vi "Terminal_Global_Pressure_system.vi"() -> ()   [LabVIEW 2014]
panel:
  out "试验单元监测参数":T1
  out "陪试单元监测参数":T2
  out "加载单元监测参数":T3
  # "报警信息"
  # "报警信息"
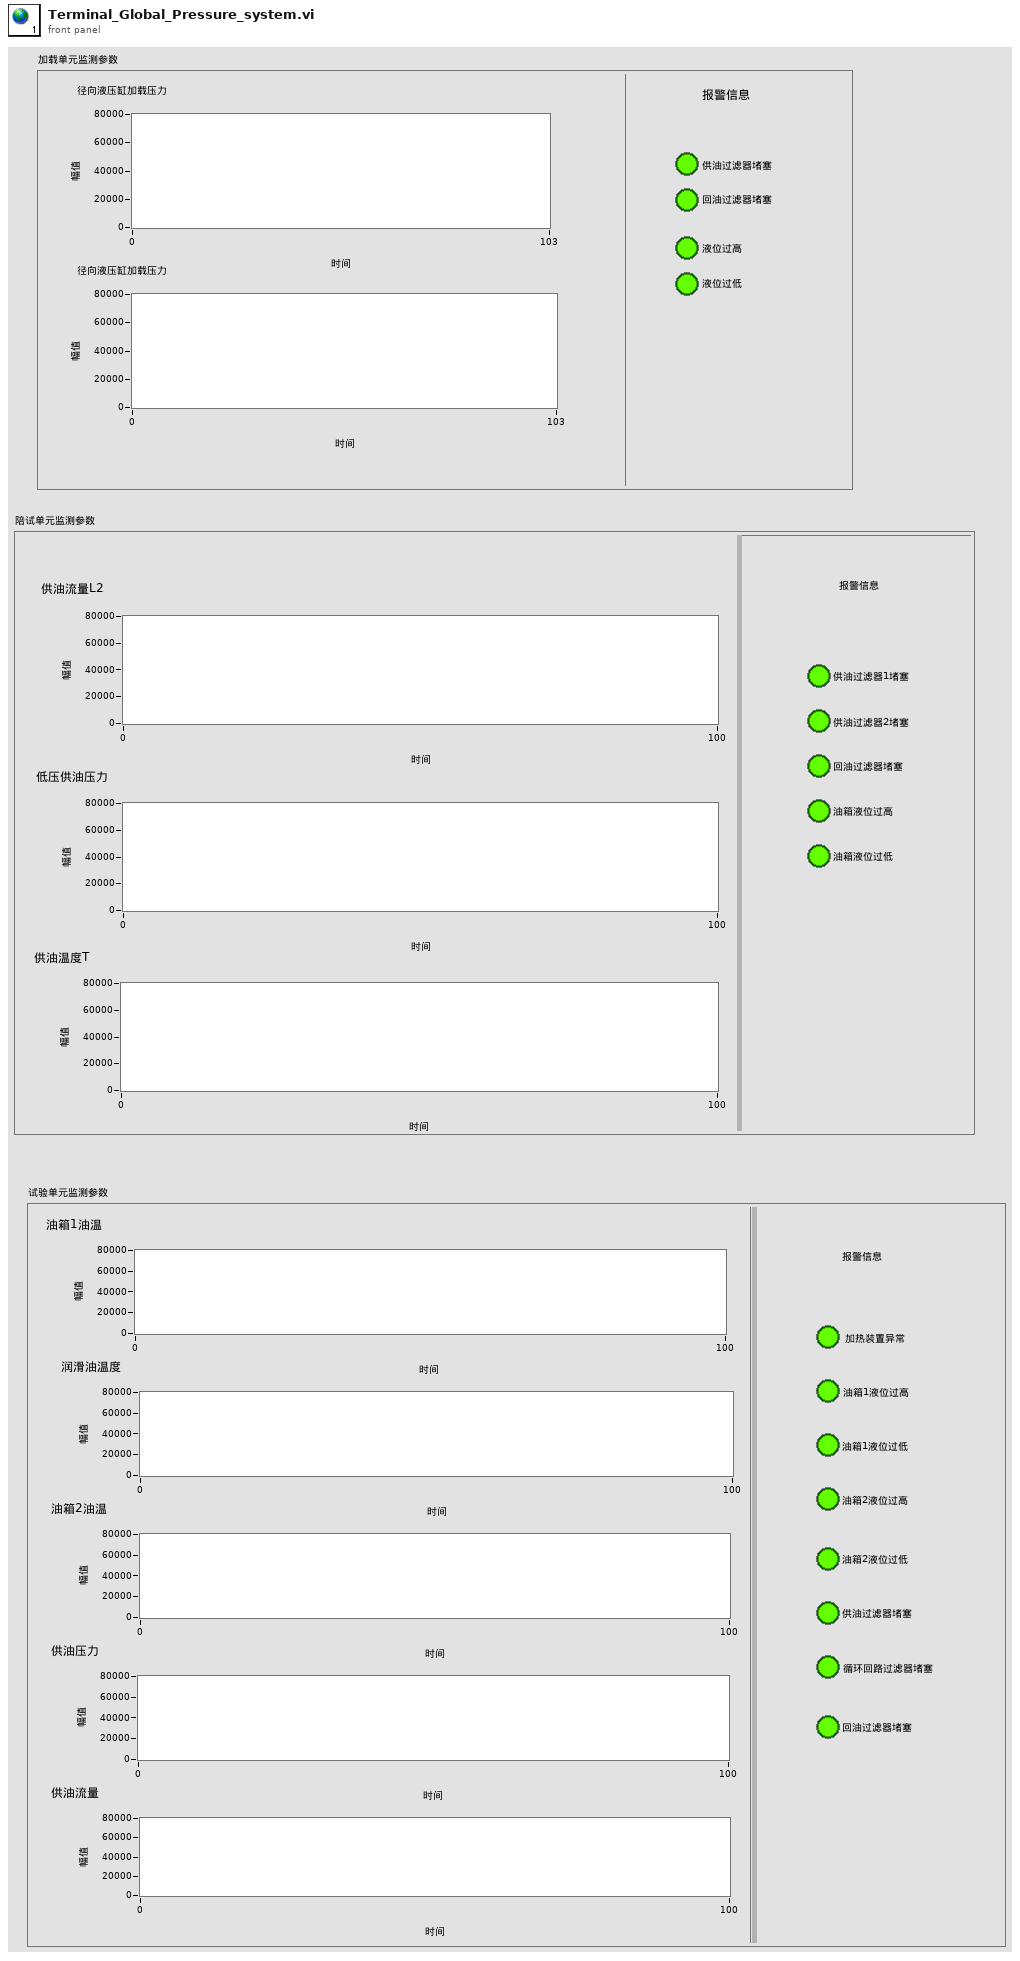
[diagram p1: front panel]
types:
  T1 = cluster{"油箱1油温 ":cluster{"油箱1油液温度":dbl, "油箱1油液温度":u16}, "润滑油温度":cluster{sgl, sgl, "润滑油温度":u16}, "油箱2油温":cluster{"油箱2油液温度":dbl, "油箱2油液温度":u16}, "径向液压缸加载压力 3":cluster{"供油压力最小值":dbl, "供油压力最大值":dbl, "试验轴承供油压力":u16}, "供油流量":cluster{sgl, sgl, "试验轴承供油流量":u16}, "报警信息":cluster{"试验轴承单元加热装置异常":bool, "试验轴承单元油箱1液位过高":bool, "试验轴承单元油箱1液位过低":bool, "试验轴承单元油箱2液位过高":bool, "试验轴承单元油箱2液位过低":bool, "试验轴承单元供油过滤器堵塞":bool, "试验轴承单元循环回路过滤器堵塞 2":bool, "试验轴承单元回油过滤器堵塞  ":bool}}
  T2 = cluster{"供油流量L2":u16, "供油压力":u16, "供油温度T":u16, "报警信息":cluster{"陪试轴承单元供油过滤器1堵塞":bool, "陪试轴承单元供油过滤器2堵塞":bool, "陪试轴承单元回油过滤器堵塞":bool, "陪试轴承单元油箱液位过高":bool, "陪试轴承单元油箱液位过低":bool}}
  T3 = cluster{"径向液压缸加载压力":u16, "轴向液压缸加载压力":u16, "报警信息":cluster{"加载单元供油过滤器堵塞":bool, "加载单元回油过滤器堵塞":bool, "加载单元液位过高":bool, "加载单元单元液位过低":bool}}
diagram:
